vi "Mood Detector (main).vi"() -> ()   [LabVIEW 2013]
uses:
  <vilib>/LabVIEW Interface for Arduino/Type Defs/Board Type.ctl
  <vilib>/LabVIEW Interface for Arduino/Type Defs/Connection Type.ctl
  <vilib>/LabVIEW Interface for Arduino/LabVIEW Interface for Arduino.lvlib
panel:
  in  "stop":bool
  out "x = y?":bool
  out "for 14k":dbl
  out "Stress":dbl
  out "Energy":dbl
  out "PSD":cluster{"f0":dbl, "df":dbl, "magnitude":dbl[]}[](graph)
  out "Mic signal":waveform(dbl)[](graph)
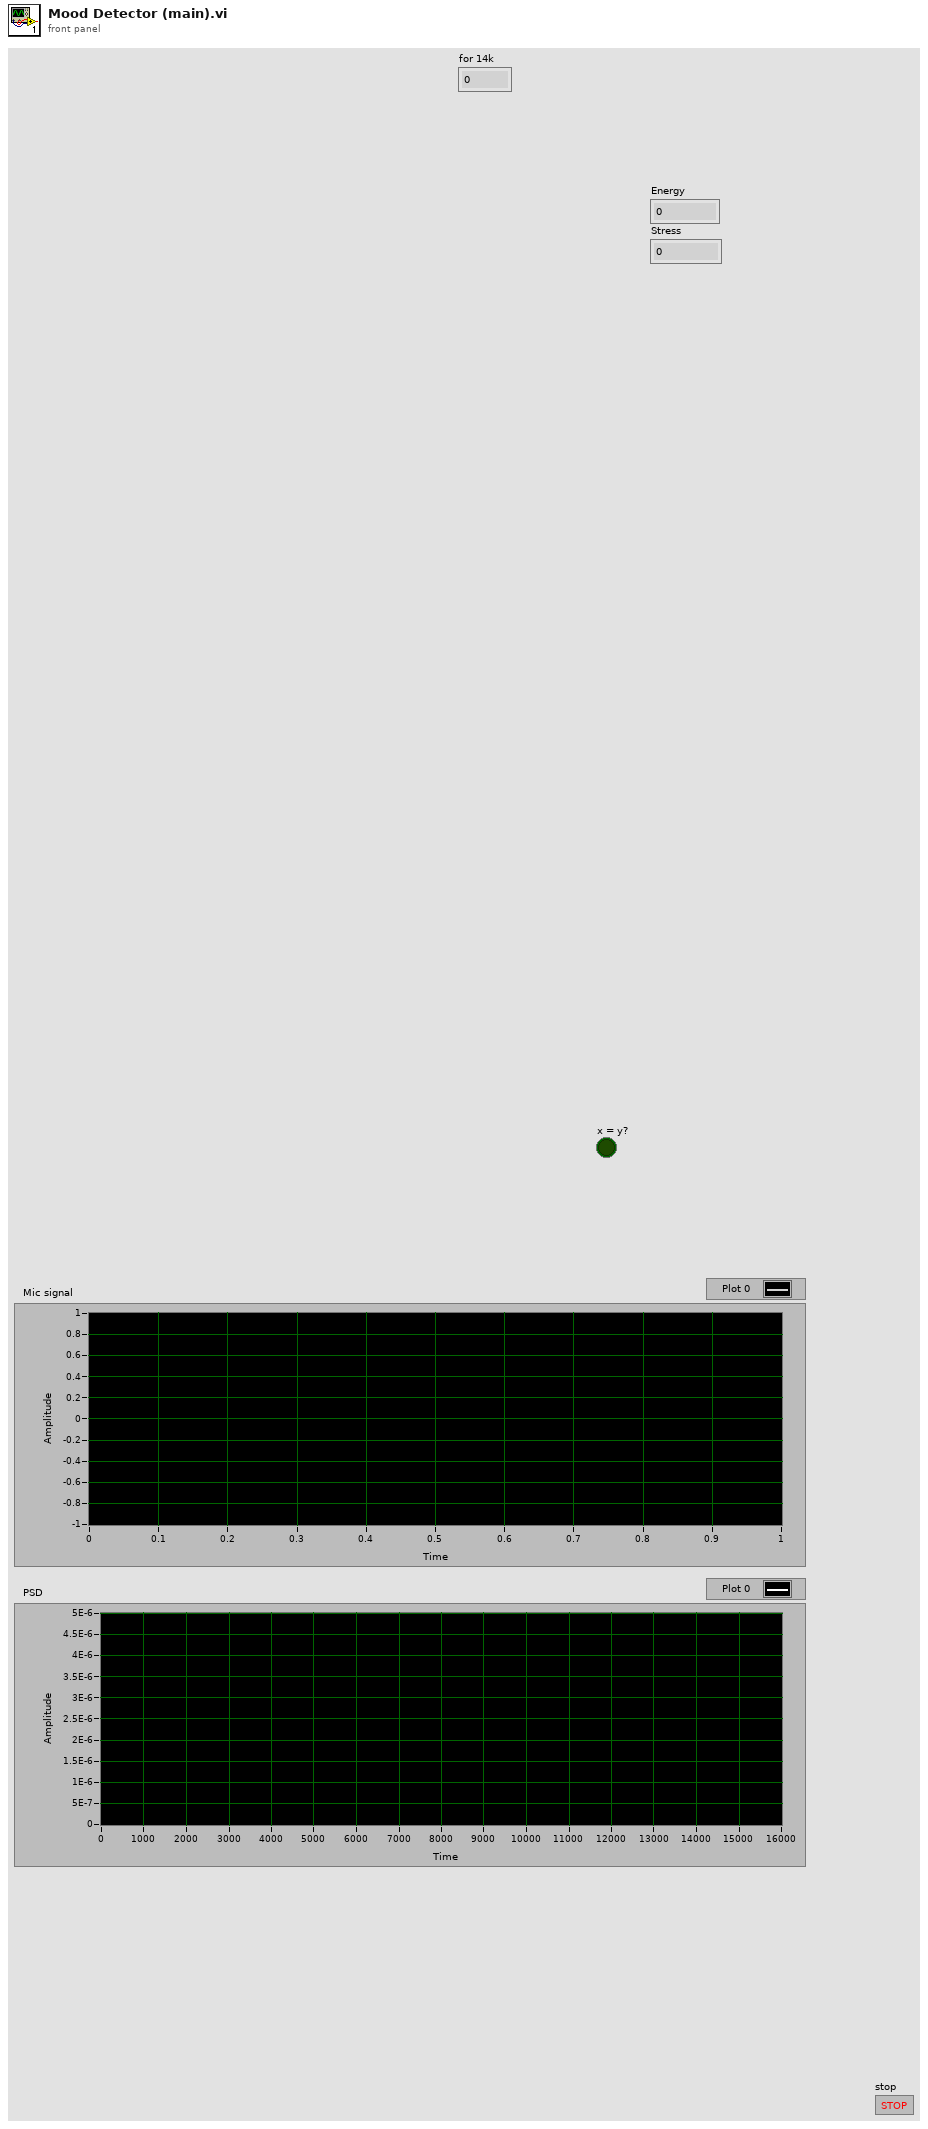
[diagram p1: front panel]
types:
  T1 = typedef "LabVIEW Interface for Arduino.lvlib/Connection Type.ctl" = enum8{"USB / Serial", "XBEE", "BlueSmirf (Bluetooth)"}
  T2 = typedef "LabVIEW Interface for Arduino.lvlib/Board Type.ctl" = enum16{"Uno", "Dimuelanove w/Atmega 328", "Mega 2560"}
  T3 = typedef "LabVIEW Interface for Arduino.lvlib/Arduino Resource.ctl" = cluster{"VISA resource":refnum<visa-resource-name>, "Board Type":T2, "Connection Type":enum8{"USB / Serial"}, "Bytes Per Packet (15)":u8}
  T4 = cluster{"Sub-Band Intensities":dbl[], "Mean Intensity":dbl}
  T5 = cluster{"Spectral Shape":cluster{"Centroid":dbl, "Rolloff":dbl, "Flux":dbl, "Zero Crossing":dbl}, "Spectral Contrast":cluster{"Valley":dbl[], "Peak":dbl[], "Average":dbl[]}}
  T6 = cluster{"Bass Instrumental Onsets":i32, "Average Strength":dbl, "Average Correlation Peak":dbl}
  T7 = cluster{"Centroid":dbl, "Rolloff":dbl, "Flux":dbl, "Zero Crossing":dbl}
  T8 = cluster{"Valley":dbl[], "Peak":dbl[], "Average":dbl[]}
  T9 = cluster{"Energy ":dbl, "Stress":dbl, dbl, "Result":dbl, "x = y?":bool}
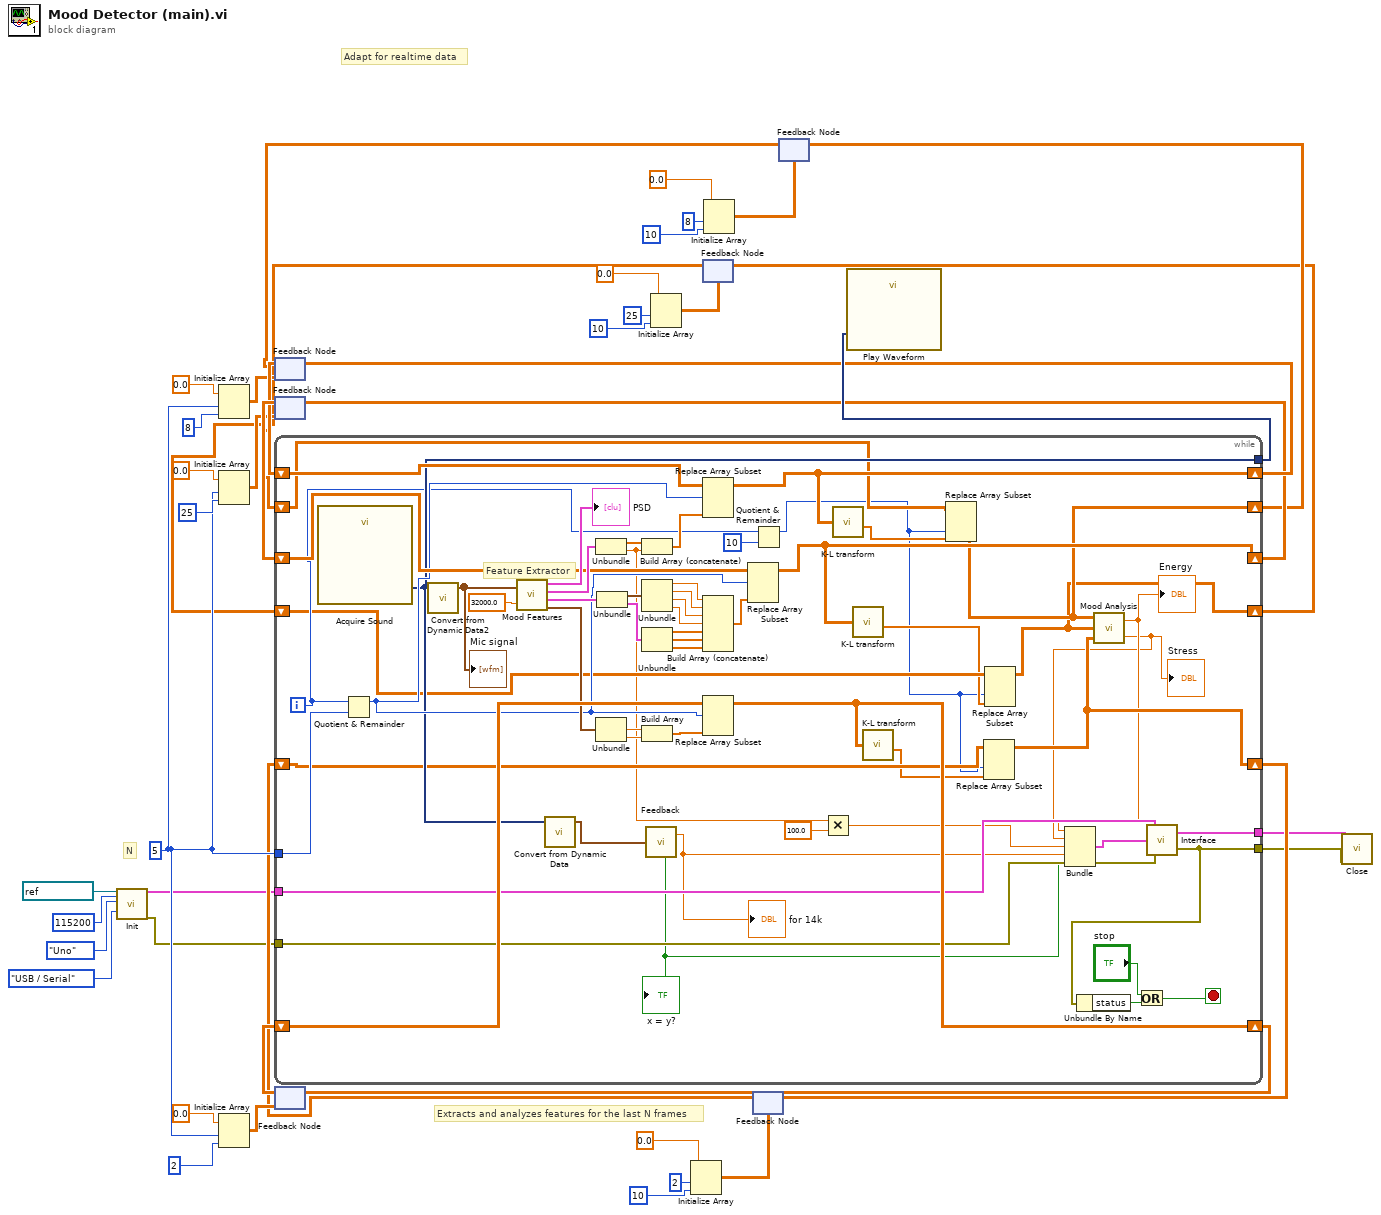
[diagram p0: block diagram]
diagram:
  w27 = 5 ("y")
  # "N"
  # "Adapt for realtime data"
  # "Extracts and analyzes features for the last N frames"
  n1 = call <vilib>:"Init.vi"("VISA resource"=refnum<visa-resource-name> "COM4", "Baud Rate (115200)"=u32 115200, "Board Type (Uno)"=Board_Type."Uno", "Connection Type (USB/Serial)"=Connection_Type."USB / Serial") -> ("Arduino Resource"=w2:T3, "error out"=w1:errorcluster)  [unwired: 14 in]
  n2 = Initialize Array(0.0 ("element"), w27, 8 ("dimension size")) -> (w38:dbl[][])
  n3 = Initialize Array(0.0 ("element"), w27, 25 ("dimension size")) -> (w34:dbl[][])
  n4 = Initialize Array(0.0 ("element"), w27, 2 ("dimension size")) -> (w35:dbl[][])
  n5 = feedback #1(w38) -> (w40:dbl[][])
  n6 = feedback #2(w34) -> (w41:dbl[][])
  n7 = feedback #3(w35) -> (w42:dbl[][])
  n8 = Initialize Array(0.0 ("element"), 25 ("dimension size"), 10 ("dimension size")) -> (w13:dbl[][])
  n9 = Initialize Array(0.0 ("element"), 2 ("dimension size"), 10 ("dimension size")) -> (w9:dbl[][])
  n10 = feedback #4(w13) -> (w19:dbl[][])
  n11 = Initialize Array(0.0 ("element"), 8 ("dimension size"), 10 ("dimension size")) -> (w21:dbl[][])
  n12 = feedback #5(w9) -> (w17:dbl[][])
  n13 = feedback #6(w21) -> (w25:dbl[][])
  n14 = while {
    tunnel: [w72] -> w43
    shift-right: [w75] -> w33
    shift-left: w40 -> [w96]
    shift-right: [w74] -> w32
    shift-left: w41 -> [w91]
    shift-right: [w73] -> w31
    shift-left: w42 -> [w82]
    tunnel: w27 -> [w76]
    shift-right: [w62] -> w26
    shift-left: w25 -> [w71]
    shift-right: [w61] -> w20
    shift-left: w19 -> [w67]
    shift-right: [w60] -> w18
    shift-left: w17 -> [w66]
    tunnel: [w58] -> w4
    tunnel: [w51] -> w3
    tunnel: w2 -> [w57]
    tunnel: w1 -> [w56]
    i -> [w68]
    stop <- w50 stop-if-true
    # "Feature Extractor"
    n15 = call "Acquire Sound"() -> ("Data"=w72:dynamicdata)  [unwired: 18 in, 1 out]
    n16 = Quotient & Remainder(x=w68, y=w76) -> (x-y*floor(x/y)=w77:i32)  [unwired: 1 out]
    n17 = call "Convert from Dynamic Data2"("Dynamic Data Type"=w72) -> ("Array of Waveform"=w101:waveform(dbl)[])  [unwired: 3 in]
    "Mic signal" <- w101
    n18 = call "Mood Features.vi"("Mic Input"=w101, "Sampling rate"=32000.0) -> ("PSD"=→"PSD":cluster{"f0":dbl, "df":dbl, "magnitude":dbl[]}[], "Intensity"=w98:T4, "Timbre"=w90:T5, "Rhythm"=w81:T6)
    n19 = call "Convert from Dynamic Data"("Dynamic Data Type"=w72) -> ("Waveform"=w59:waveform(dbl))  [unwired: 3 in]
    n20 = Unbundle(w98) -> ("Sub-Band Intensities"=w97:dbl[], "Mean Intensity"=w54:dbl)
    n21 = Unbundle(w81) -> ("Average Strength"=w80:dbl, "Average Correlation Peak"=w79:dbl)  [unwired: 1 out]
    n22 = Unbundle(w90) -> ("Spectral Shape"=w89:T7, "Spectral Contrast"=w88:T8)
    n23 = Build Array (concatenate)(w97, w54) -> (w95:dbl[])
    n24 = Unbundle(w89) -> ("Centroid"=w93:dbl, "Rolloff"=w94:dbl, "Flux"=w87:dbl, "Zero Crossing"=w86:dbl)
    n25 = Unbundle(w88) -> ("Valley"=w85:dbl[], "Peak"=w84:dbl[], "Average"=w83:dbl[])
    n26 = Build Array(w80, w79) -> (w78:dbl[])
    n27 = call "Feedback.vi"("time signal"=w59) -> ("Result"=w45:dbl, "x = y?"=w47:bool)
    "for 14k" <- w45
    "x = y?" <- w47
    n28 = Replace Array Subset(array=w96, new element=w95, index (row)=w77) -> (w75:dbl[][])  [unwired: 1 in]
    n29 = Build Array (concatenate)(w93, w94, w87, w86, w85, w84, w83) -> (w92:dbl[])
    n30 = Replace Array Subset(array=w82, new element=w78, index (row)=w77) -> (w73:dbl[][])  [unwired: 1 in]
    n31 = Replace Array Subset(array=w91, new element=w92, index (row)=w77) -> (w74:dbl[][])  [unwired: 1 in]
    n32 = Quotient & Remainder(x=w68, y=10) -> (x-y*floor(x/y)=w63:i32)  [unwired: 1 out]
    n33 = Multiply(x=w54, y=100.0) -> (x*y=w46:dbl)
    n34 = call "K-L transform.vi"("Dataset"=w75) -> ("Feature Vector"=w70:dbl[])  [unwired: 3 out]
    n35 = call "K-L transform.vi"("Dataset"=w74) -> ("Feature Vector"=w65:dbl[])  [unwired: 3 out]
    n36 = call "K-L transform.vi"("Dataset"=w73) -> ("Feature Vector"=w64:dbl[])  [unwired: 3 out]
    n37 = Replace Array Subset(array=w71, new element=w70, index (col)=w63) -> (w62:dbl[][])  [unwired: 1 in]
    n38 = Replace Array Subset(array=w66, new element=w64, index (col)=w63) -> (w60:dbl[][])  [unwired: 1 in]
    n39 = Replace Array Subset(array=w67, new element=w65, index (col)=w63) -> (w61:dbl[][])  [unwired: 1 in]
    n40 = call "Mood Analysis.vi"("Rhythm"=w60, "Timbre"=w61, "Intensity"=w62) -> ("Stress"=w48:dbl, "Energy"=w49:dbl)
    "Energy" <- w49
    "Stress" <- w48
    n41 = Bundle("Energy"=w49, "Stress"=w48, w46, "Result"=w45, "x = y?"=w47) -> (w44:T9)  [unwired: 1 in]
    n42 = call "Interface.vi"("error in"=w56, "Values"=w44, "Arduino Resource"=w57) -> ("error out"=w51:errorcluster, "Arduino Resource"=w58:T3)
    n43 = Unbundle By Name(w51) -> ("status"=w53:bool)
    n44 = Or(x="stop", y=w53) -> (x .or. y?=w50:bool)
  }
  n45 = feedback-in #1(w33) -> ()
  n46 = feedback-in #2(w32) -> ()
  n47 = feedback-in #3(w31) -> ()
  n48 = feedback-in #4(w20) -> ()
  n49 = feedback-in #5(w18) -> ()
  n50 = feedback-in #6(w26) -> ()
  n51 = call "Play Waveform"("Data"=w43) -> ()  [unwired: 18 in, 1 out]
  n52 = call <vilib>:"Close.vi"("Arduino Resource"=w4, "error in"=w3) -> ()  [unwired: 13 in, 1 out]
